vi "ToteFirstAuton.vi"() -> ()   [LabVIEW 2014]
uses:
  <vilib>/Rock Robotics/WPI/Relay/WPI_RelayValue.ctl
  Robot Values.vi
panel:
  in  "turn output range":cluster{"output high":dbl, "output low":dbl}={"output high"=0.4, "output low"=-0.4} {"output low" format="%.2f"; "output high" format="%.2f"}
  in  "PID Turn  gains":T1={"proportional gain (Kc)"=0.05, "integral time (Ti, min)"=0.01, "derivative time (Td, min)"=0.0} {"derivative time (Td, min)" format="%.3f"; "integral time (Ti, min)" format="%.3f"; "proportional gain (Kc)" format="%.3f"}
  in  "Average gains":T1
  in  "output range":cluster{"output high":dbl, "output low":dbl}
  out "Total totes":i32
  out "Totes grabed":i32
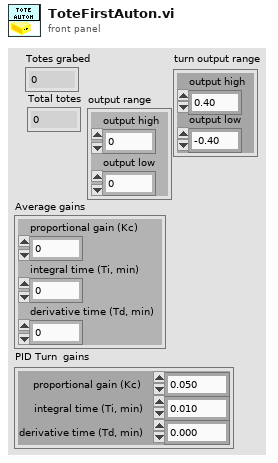
[diagram p1: front panel]
types:
  T1 = cluster{"proportional gain (Kc)":dbl, "integral time (Ti, min)":dbl, "derivative time (Td, min)":dbl}
  T2 = enum16{"Nothing", "Start", "Push", "Finish", "Turn", "Stack"}
  T3 = typedef "WPI_RelayValue.ctl" = enum16{"Off", "On", "Forward", "Reverse"}
  T4 = cluster{"Tracking Tote?":bool, "ToteRightSpeed":dbl, "ToteLeftSpeed":dbl, "Drive Encoder reset":bool, "Right Wheel \n(Cm)":dbl, "Left Wheel \n(Cm)":dbl}
  T5 = cluster{"Lift Position":i32, "Lift Speed Override":dbl, "OverrideTele?":bool, "OverrideDash":bool}
  T6 = cluster{"Lift Encoder Height Right (cm)":dbl, "Lift Encoder Height Left (cm)":dbl, "Right Prox":bool, "Left Prox":bool, "Gyro Angle":dbl, "Gyro anglar rate":dbl, "Gyro Reset":bool}
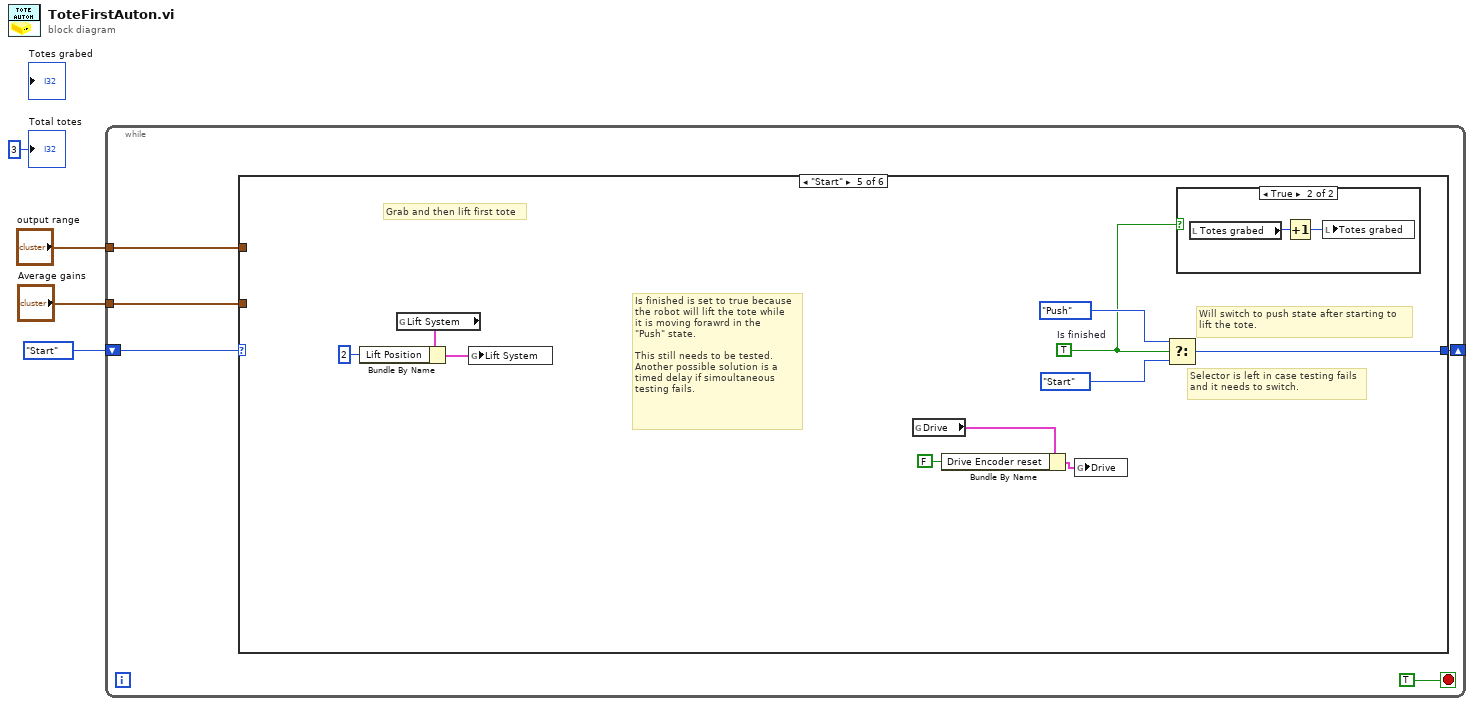
[diagram p0: block diagram]
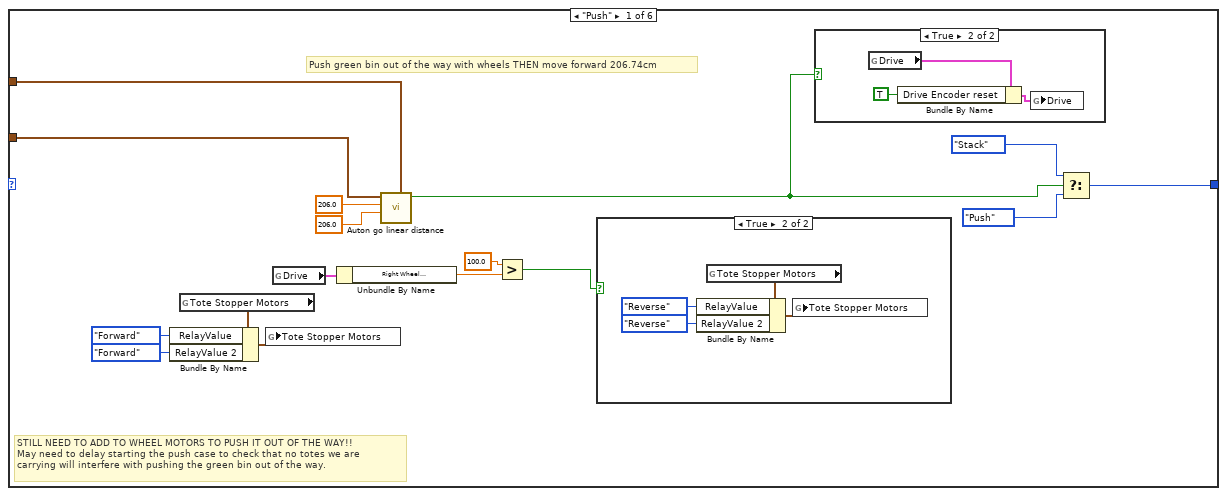
[diagram p2: hidden frame]
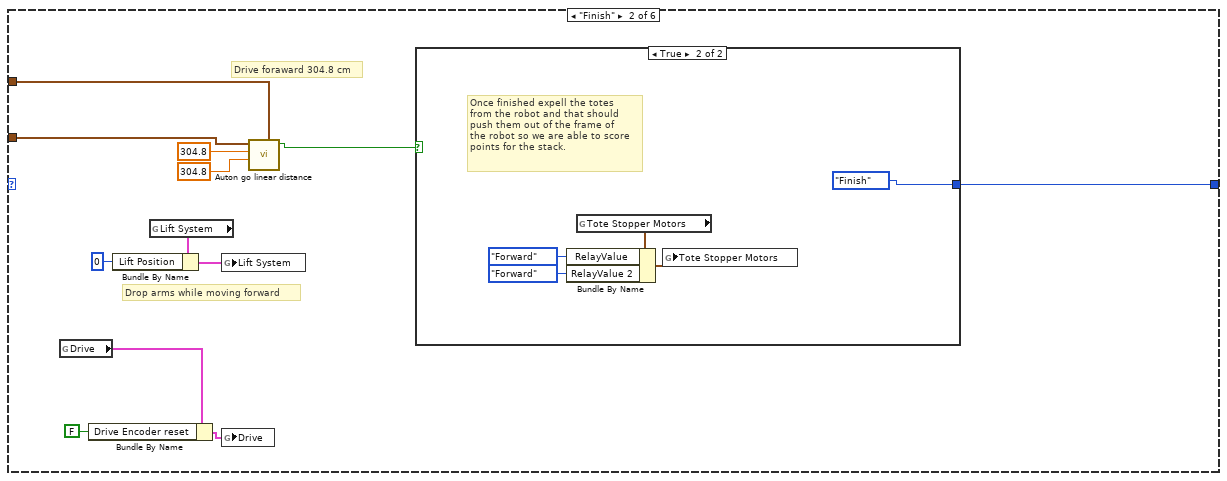
[diagram p5: hidden frame]
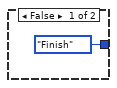
[diagram p6: hidden frame]
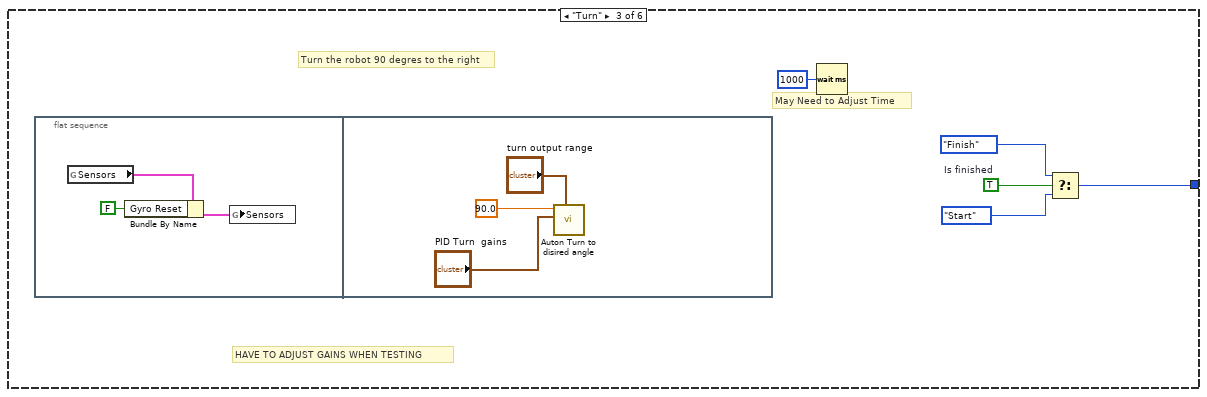
[diagram p7: hidden frame]
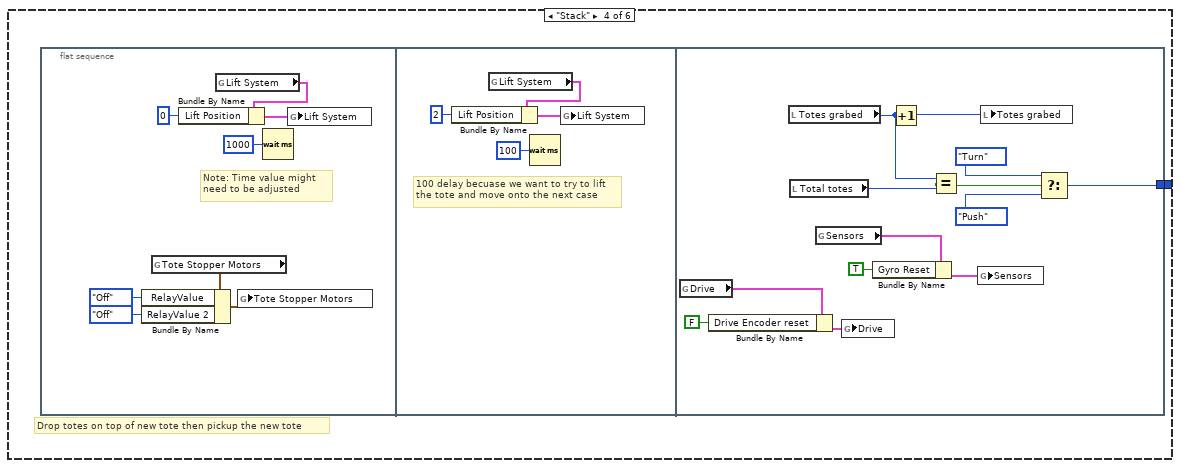
[diagram p8: hidden frame]
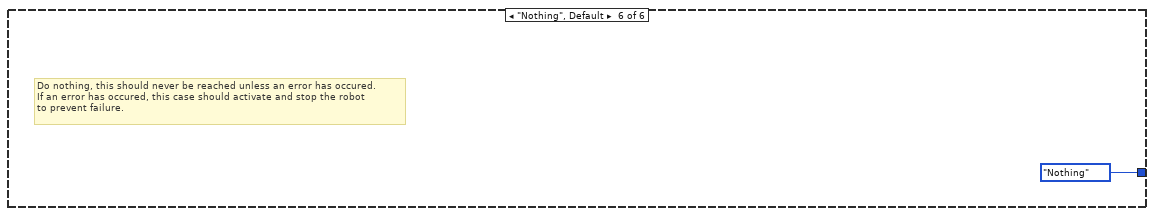
[diagram p10: hidden frame]
diagram:
  n1 = while {
    shift-right: [w8] -> _
    shift-left: T2."Start" -> [w9]
    tunnel: "Average gains" -> [w6]
    tunnel: "output range" -> [w5]
    stop <- TRUE stop-if-true
    n2 = case shown="\"Start\"" w9 {
      tunnel: [w23 w36 w52 w62 w95 T2."Nothing"] -> w8
      tunnel: w6 -> [w21 w41 _ _ _ _]
      tunnel: w5 -> [w22 w42 _ _ _ _]
      frame "Push" {
        # "STILL NEED TO ADD TO WHEEL MOTORS TO PUSH IT OUT OF THE WAY!!\nMay need to delay starting the push case to check that no totes we are \ncarrying will interfere with pushing the green bin out of the way."
        # "Push green bin out of the way with wheels THEN move forward 206.74cm"
        n3 = global read "Robot Values.vi" "Tote Stopper Motors"() -> (w18:cluster{"RelayValue":T3, "RelayValue 2":T3})
        n4 = Bundle By Name(cluster=w18, "RelayValue"=WPI_RelayValue."Forward", "RelayValue 2"=WPI_RelayValue."Forward") -> (w19:cluster{"RelayValue":T3, "RelayValue 2":T3})
        n5 = global write "Robot Values.vi" "Tote Stopper Motors"(w19) -> ()
        n6 = global read "Robot Values.vi" "Drive"() -> (w13:T4)
        n7 = Unbundle By Name(w13) -> ("Right Wheel \n(Cm)"=w11:dbl)
        n8 = call "Auton go linear distance.vi"("Average gains"=w21, "PID setpoint"=206.0, "Goal"=206.0, "output range"=w22) -> ("Done?"=w15:bool)  [unwired: 4 in]
        n9 = Greater?(x=100.0, y=w11) -> (0:w10:bool)
        n10 = case shown="True" w10 {
          frame False {
          }
          frame True {
            n11 = global read "Robot Values.vi" "Tote Stopper Motors"() -> (w27:cluster{"RelayValue":T3, "RelayValue 2":T3})
            n12 = Bundle By Name(cluster=w27, "RelayValue"=WPI_RelayValue."Reverse", "RelayValue 2"=WPI_RelayValue."Reverse") -> (w26:cluster{"RelayValue":T3, "RelayValue 2":T3})
            n13 = global write "Robot Values.vi" "Tote Stopper Motors"(w26) -> ()
          }
        }
        n14 = case shown="True" w15 {
          frame False {
          }
          frame True {
            n15 = global read "Robot Values.vi" "Drive"() -> (w31:T4)
            n16 = Bundle By Name(cluster=w31, "Drive Encoder reset"=TRUE) -> (w32:T4)
            n17 = global write "Robot Values.vi" "Drive"(w32) -> ()
          }
        }
        n18 = Select(t=T2."Stack", s=w15, f=T2."Push") -> (s? t:f=w23:T2)
      }
      frame "Finish" {
        # "Drop arms while moving forward"
        # "Drive foraward 304.8 cm"
        n19 = global read "Robot Values.vi" "Drive"() -> (w38:T4)
        n20 = Bundle By Name(cluster=w38, "Drive Encoder reset"=FALSE) -> (w39:T4)
        n21 = global read "Robot Values.vi" "Lift System"() -> (w34:T5)
        n22 = Bundle By Name(cluster=w34, "Lift Position"=0) -> (w35:T5)
        n23 = global write "Robot Values.vi" "Lift System"(w35) -> ()
        n24 = global write "Robot Values.vi" "Drive"(w39) -> ()
        n25 = call "Auton go linear distance.vi"("Average gains"=w41, "PID setpoint"=304.8, "Goal"=304.8, "output range"=w42) -> ("Done?"=w40:bool)  [unwired: 4 in]
        n26 = case shown="True" w40 {
          tunnel: [T2."Finish" T2."Finish"] -> w36
          frame False {
          }
          frame True {
            # "Once finished expell the totes\nfrom the robot and that should\npush them out of the frame of\nthe robot so we are able to score\npoints for the stack."
            n27 = global read "Robot Values.vi" "Tote Stopper Motors"() -> (w48:cluster{"RelayValue":T3, "RelayValue 2":T3})
            n28 = Bundle By Name(cluster=w48, "RelayValue"=WPI_RelayValue."Forward", "RelayValue 2"=WPI_RelayValue."Forward") -> (w49:cluster{"RelayValue":T3, "RelayValue 2":T3})
            n29 = global write "Robot Values.vi" "Tote Stopper Motors"(w49) -> ()
          }
        }
      }
      frame "Turn" {
        w53 = TRUE  # Is finished
        # "May Need to Adjust Time"
        # "HAVE TO ADJUST GAINS WHEN TESTING"
        # "Turn the robot 90 degres to the right"
        n30 = flat-sequence {
          frame #0 {
            n31 = global read "Robot Values.vi" "Sensors"() -> (w57:T6)
            n32 = Bundle By Name(cluster=w57, "Gyro Reset"=FALSE) -> (w56:T6)
            n33 = global write "Robot Values.vi" "Sensors"(w56) -> ()
          }
          frame #1 {
            n34 = call "Auton Turn to disired angle.vi"("Power output range"="turn output range", "PID Turn  gains"="PID Turn  gains", "Angle setpoint"=90.0) -> ()  [unwired: 9 in]
          }
        }
        n35 = Wait (ms)(milliseconds to wait=u32 1000) -> ()  [unwired: 1 out]
        n36 = Select(t=T2."Finish", s=w53, f=T2."Start") -> (s? t:f=w52:T2)
      }
      frame "Stack" {
        # "Drop totes on top of new tote then pickup the new tote"
        n37 = flat-sequence {
          tunnel: [w87] -> w62
          frame #0 {
            # "Note: Time value might \nneed to be adjusted"
            n38 = global read "Robot Values.vi" "Tote Stopper Motors"() -> (w65:cluster{"RelayValue":T3, "RelayValue 2":T3})
            n39 = Bundle By Name(cluster=w65, "RelayValue"=WPI_RelayValue."Off", "RelayValue 2"=WPI_RelayValue."Off") -> (w66:cluster{"RelayValue":T3, "RelayValue 2":T3})
            n40 = global read "Robot Values.vi" "Lift System"() -> (w69:T5)
            n41 = Bundle By Name(cluster=w69, "Lift Position"=0) -> (w68:T5)
            n42 = global write "Robot Values.vi" "Tote Stopper Motors"(w66) -> ()
            n43 = Wait (ms)(milliseconds to wait=u32 1000) -> ()  [unwired: 1 out]
            n44 = global write "Robot Values.vi" "Lift System"(w68) -> ()
          }
          frame #1 {
            # "100 delay becuase we want to try to lift\nthe tote and move onto the next case"
            n45 = global read "Robot Values.vi" "Lift System"() -> (w73:T5)
            n46 = Bundle By Name(cluster=w73, "Lift Position"=2) -> (w74:T5)
            n47 = Wait (ms)(milliseconds to wait=u32 100) -> ()  [unwired: 1 out]
            n48 = global write "Robot Values.vi" "Lift System"(w74) -> ()
          }
          frame #2 {
            n49 = global read "Robot Values.vi" "Drive"() -> (w76:T4)
            n50 = Bundle By Name(cluster=w76, "Drive Encoder reset"=FALSE) -> (w77:T4)
            n51 = local read "Totes grabed"() -> (w86:i32)
            n52 = local read "Total totes"() -> (w84:i32)
            n53 = global read "Robot Values.vi" "Sensors"() -> (w79:T6)
            n54 = global write "Robot Values.vi" "Drive"(w77) -> ()
            n55 = Bundle By Name(cluster=w79, "Gyro Reset"=TRUE) -> (w80:T6)
            n56 = Increment(x=w86) -> (x+1=w85:i32)
            n57 = Equal?(x=w85, y=w84) -> (x = y?=w82:bool)
            n58 = global write "Robot Values.vi" "Sensors"(w80) -> ()
            n59 = local write "Totes grabed"(w85) -> ()
            n60 = Select(t=T2."Turn", s=w82, f=T2."Push") -> (s? t:f=w87:T2)
          }
        }
      }
      frame "Start" {
        w94 = TRUE  # Is finished
        # "Selector is left in case testing fails\nand it needs to switch."
        # "Will switch to push state after starting to\nlift the tote."
        # "Is finished is set to true because\nthe robot will lift the tote while\nit is moving forawrd in the\n\"Push\" state.\n\nThis still needs to be tested.\nAnother possible solution is a\ntimed delay if simoultaneous\ntesting fails."
        # "Grab and then lift first tote"
        n61 = global read "Robot Values.vi" "Lift System"() -> (w92:T5)
        n62 = Bundle By Name(cluster=w92, "Lift Position"=2) -> (w93:T5)
        n63 = global write "Robot Values.vi" "Lift System"(w93) -> ()
        n64 = global read "Robot Values.vi" "Drive"() -> (w89:T4)
        n65 = Bundle By Name(cluster=w89, "Drive Encoder reset"=FALSE) -> (w90:T4)
        n66 = global write "Robot Values.vi" "Drive"(w90) -> ()
        n67 = Select(t=T2."Push", s=w94, f=T2."Start") -> (s? t:f=w95:T2)
        n68 = case shown="True" w94 {
          frame False {
          }
          frame True {
            n69 = local read "Totes grabed"() -> (w99:i32)
            n70 = Increment(x=w99) -> (x+1=w98:i32)
            n71 = local write "Totes grabed"(w98) -> ()
          }
        }
      }
      frame "Nothing", Default {
        # "Do nothing, this should never be reached unless an error has occured.\nIf an error has occured, this case should activate and stop the robot\nto prevent failure."
      }
    }
  }
  "Total totes" <- 3 ("Total totes")
